vi "GetExternalInterfaces.vi"(8 "ErrorIn":errorcluster, 11 "ReferenceIn":refnum<class "DemoApplication.lvclass">) -> (0 "ErrorOut":errorcluster, 2 "ExternalInterfaces":T1[](array[typedef]), 3 "ReferenceOut":refnum<class "DemoApplication.lvclass">)   [LabVIEW 2021, in "DemoApplication.lvclass"]
uses:
  DemoApplication.lvclass
  .Externals/Library_TAF_Support/ClusterArrayConversion/BundledArray.ctl
  ec6bb0d8-241c-4bf6-bd1f-df29f73ad419.vi
  <vilib>/Utility/Data Type/Get Cluster Information.vi
  <vilib>/Utility/Data Type/Get Type Information.vi
  .Externals/Library_TAF_ApplicationFramework/MasterGUI/MasterGUI.lvclass
  DemoApplication.lvclass/DemoApplication.ctl
  .Externals/Library_TAF_Support/ClusterArrayConversion/ClusterArrayConversion.lvlib
  IInterface/IInterface.lvclass
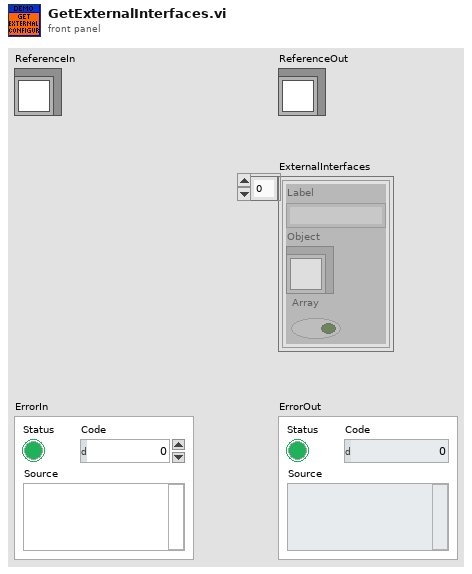
[diagram p1: front panel]
types:
  T1 = typedef "ClusterArrayConversion.lvlib/BundledArray.ctl" = cluster{"Label":string, "Object":refnum<class>, "Array":bool}
  T2 = typedef "DemoApplication.lvclass/ObjectAttributes.ctl" = cluster{"Interfaces":cluster{"Authorizer":refnum<class "IAuthorization.lvclass">, "TextViewer":refnum<class "ITAFTextViewer.lvclass">, "ApplicationConfiguration":refnum<class "IApplicationConfiguration.lvclass">, "Tracer":refnum<class "IFrontPanel.lvclass">}, "Persistent":cluster{"MenuEnables":cluster{"MenuTag":string, "MenuExpression":string}[], "TextDockSubPanelName":string}}
  T3 = cluster{"Authorizer":refnum<class "IAuthorization.lvclass">, "TextViewer":refnum<class "ITAFTextViewer.lvclass">, "ApplicationConfiguration":refnum<class "IApplicationConfiguration.lvclass">, "Tracer":refnum<class "IFrontPanel.lvclass">}
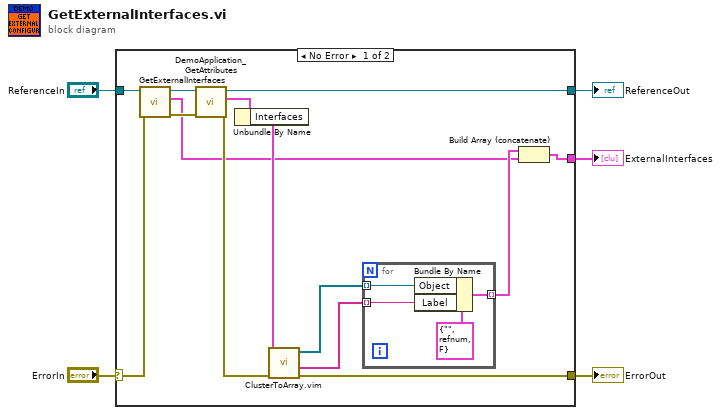
[diagram p0: block diagram]
diagram:
  n1 = case shown="No Error" "ErrorIn" {
    selector: "ErrorIn" -> [w19 w25]
    tunnel: [w17 w25] -> w4
    tunnel: [w14 w24] -> w2
    tunnel: "ReferenceIn" -> [w8 w24]
    tunnel: [w10 _] -> w1
    frame No Error {
      n2 = call-parent "GetExternalInterfaces.vi"("ErrorIn"=w19, "ReferenceIn"=w8) -> ("ErrorOut"=w16:errorcluster, "ExternalInterfaces"=w6:T1[], "ReferenceOut"=w7:refnum<class "DemoApplication.lvclass">)  [unwired: 7 in]
      n3 = call "DemoApplication_GetAttributes.vi"("ErrorIn"=w16, "ReferenceIn"=w7) -> ("ErrorOut"=w18:errorcluster, "Data"=w15:T2, "ReferenceOut"=w14:refnum<class "DemoApplication.lvclass">)  [unwired: 6 in, 1 out]
      n4 = Unbundle By Name(w15) -> ("Interfaces"=w13:T3)
      n5 = call "ClusterToArray.vim"("ErrorIn"=w18, "Cluster"=w13) -> ("ErrorOut"=w17:errorcluster, "Labels"=w11:string[], "ArrayOfElements"=w12:refnum<class "IInterface.lvclass">[])  [unwired: 7 in]
      n6 = for {
        tunnel: w12 -> [w22] mode=indexing
        tunnel: w11 -> [w21] mode=indexing
        tunnel: [w20] -> w9 mode=indexing
        n7 = Bundle By Name(cluster=T1 {"Label"="", "Object"=refnum, "Array"=FALSE} ("ExternalInterface"), "Object"=w22, "Label"=w21) -> (w20:T1)
      }
      n8 = Build Array (concatenate)(w9, w6) -> (w10:T1[])
    }
    frame Error {
    }
  }
  "ErrorOut" <- w4
  "ReferenceOut" <- w2
  "ExternalInterfaces" <- w1
